vi "IRH1-2T_ConstructiveHeuristic.vi"(9 "Initial Construction Heursitic":T1, 10 "Scheduler":T2(ring)=enum."Non Delay Scheduler", 11 "Proocessing Times MxJ":u16[][](array[numeric])=[[1, 69, 192, 47, 292, 28, 166, 205], [146, 96, 177, 62, 37, 145, 3, 334], [99, 182, 133, 113, 9, 239, 27, 198], [159, 182, 132, 158, 183, 38, 142, 6], [92, 63, 114, 144, 180, 199, 136, 72], [119, 31, 9, 163, 139, 158, 350, 31], [46, 30, 59, 290, 156, 90, 175, 154], [338, 347, 184, 23, 4, 103, 1, 0]]) -> (1 "Due Dates":u16[](array[numeric]), 2 "Total Tardiness":i32, 3 "IRH2T Schedule Out":u16[](array[numeric]))   [LabVIEW 2013]
uses:
  Initial Construction Heuristic.ctl
  Classes/GanntChart.lvclass
panel:
  in  "Proocessing Times (8x8)":u16[][](array[numeric])=[[1, 69, 192, 47, 292, 28, 166, 205], [146, 96, 177, 62, 37, 145, 3, 334], [99, 182, 133, 113, 9, 239, 27, 198], [159, 182, 132, 158, 183, 38, 142, 6], [92, 63, 114, 144, 180, 199, 136, 72], [119, 31, 9, 163, 139, 158, 350, 31], [46, 30, 59, 290, 156, 90, 175, 154], [338, 347, 184, 23, 4, 103, 1, 0]]
  out "Machine Completion Times":u16[](array[numeric])
  out "Completion Times":u16[][](array[numeric])
  out "Job Completion Times":i32[](array[numeric])
  out "String":string
  out "LPT Array":i32[](array[numeric])
  # "1, 69, 192, 47, 292, 28, 166, 205], \n[146, 96, 177, 62, 37, 145, 3, 334], \n[99, 182, 133, 113, 9, 239, 27, 198], \n[159, 182, 132, 158, 183, 38, 142, 6], \n[92, 63, 114, 144, 180, 199, 136, 72], \n[119, 31, 9, 163, 139, 158, 350, 31], \n[46, 30, 59, 290, 156, 90, 175, 154], \n[338, 347, 184, 23, 4, 103, 1, 0]]"
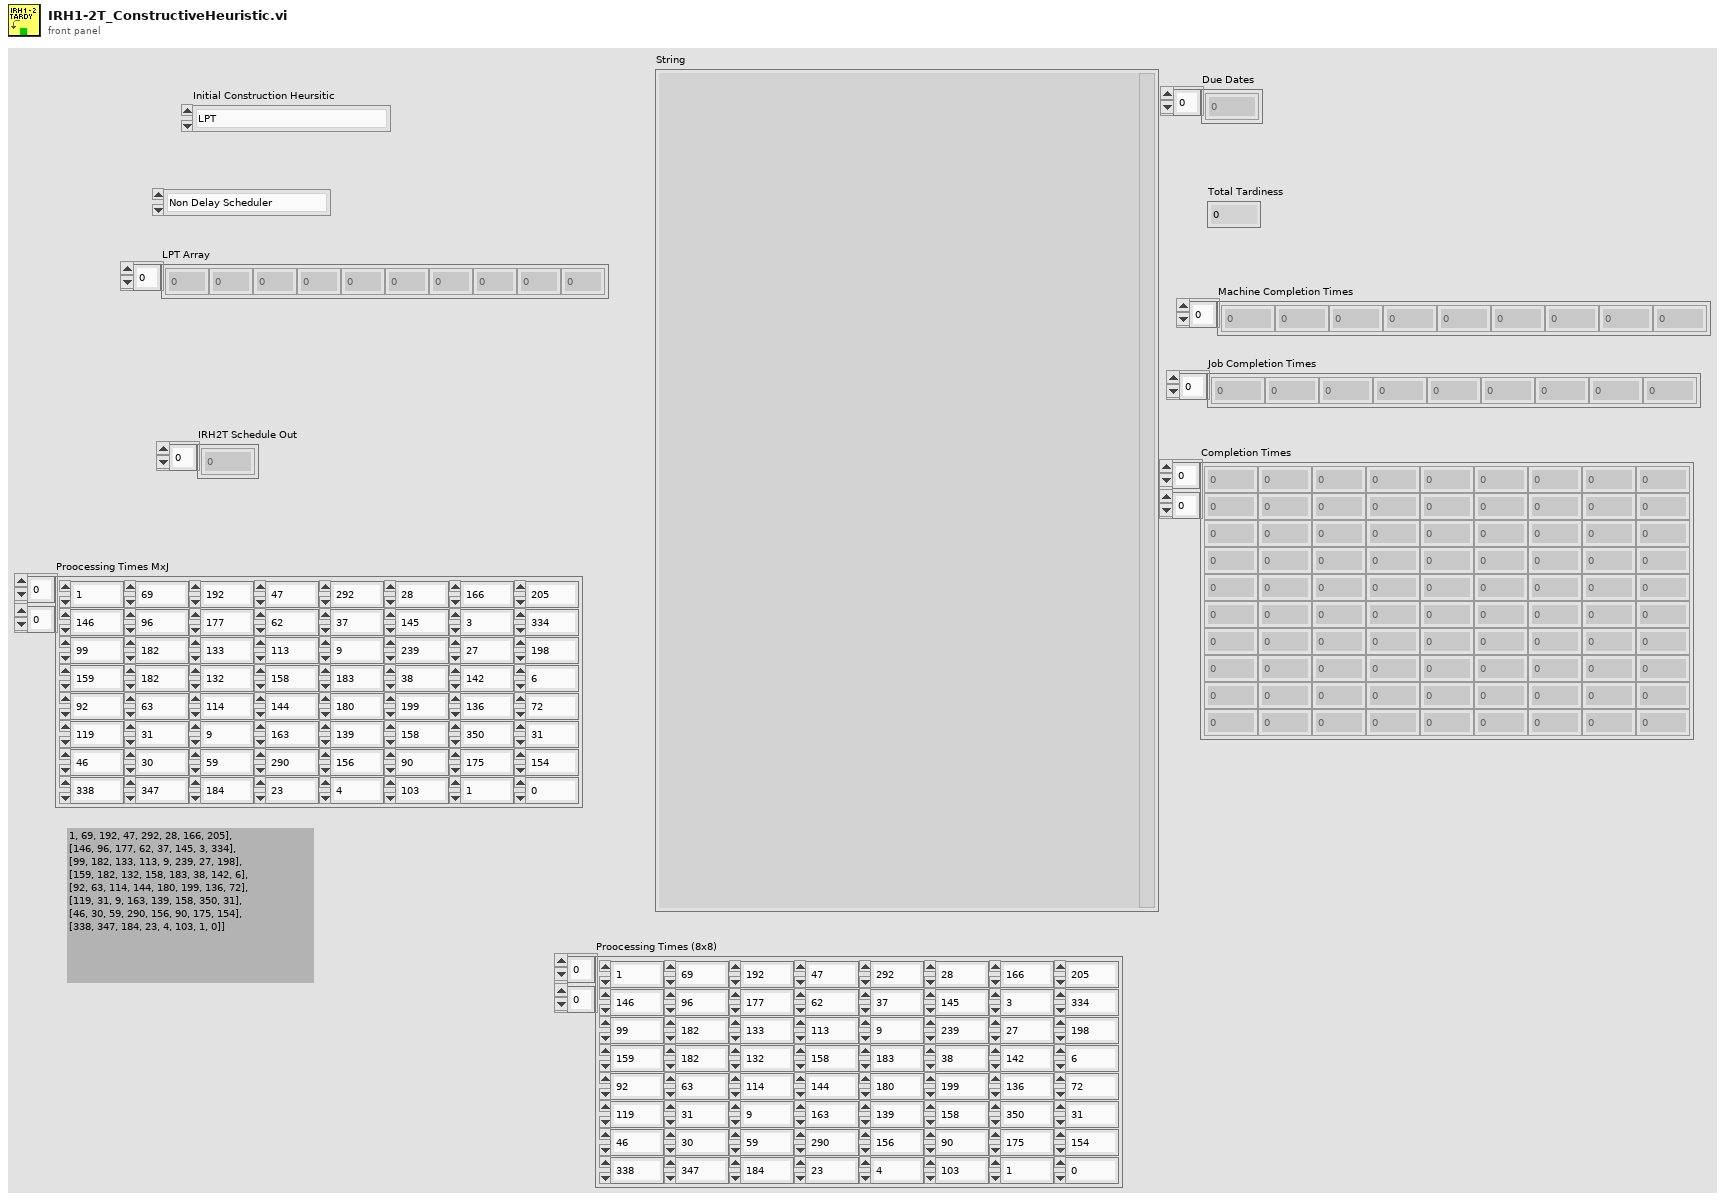
[diagram p1: front panel]
types:
  T1 = typedef "Initial Construction Heuristic.ctl" = enum16{"LPT", "SPT", "EDD"}
  T2 = enum16{"Semi Active Scheduler", "Non Delay Scheduler"}
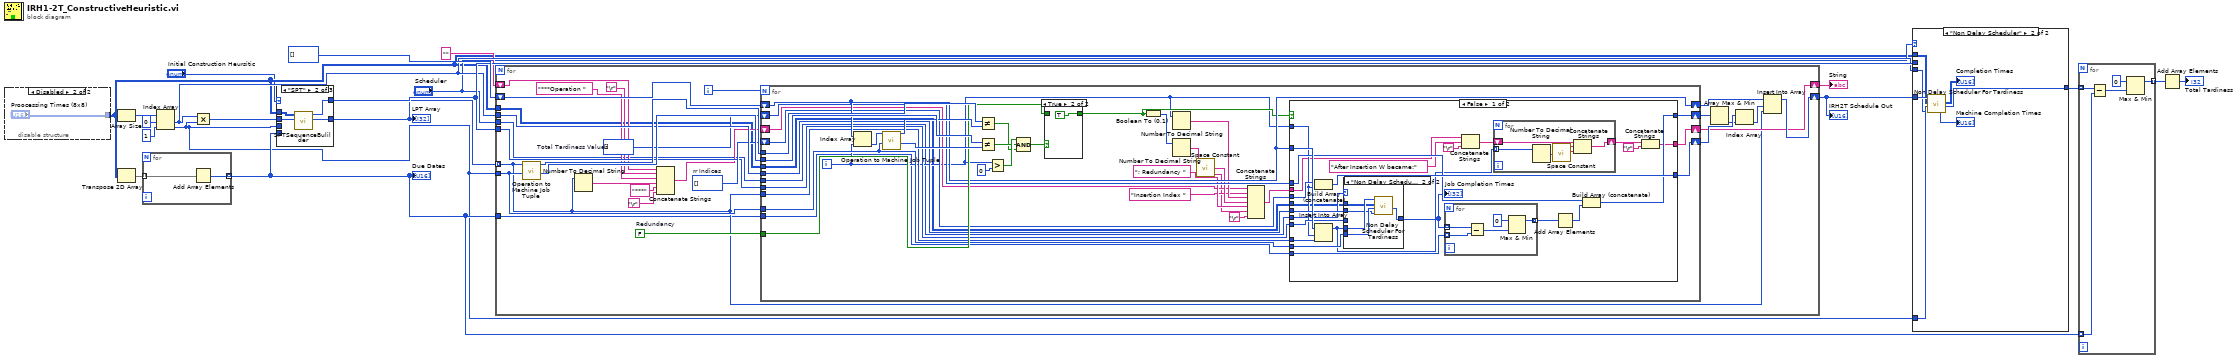
[diagram p0: block diagram]
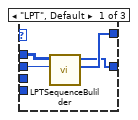
[diagram p2: hidden frame]
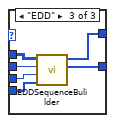
[diagram p3: hidden frame]
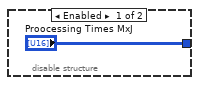
[diagram p4: hidden frame]
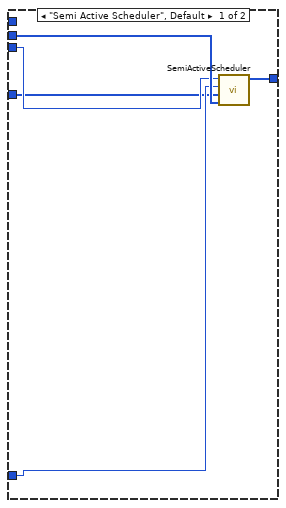
[diagram p5: hidden frame]
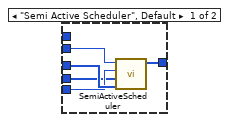
[diagram p6: hidden frame]
diagram:
  n1 = disable-structure shown="Disabled" {
    disable-tunnel: ["Proocessing Times MxJ" "Proocessing Times (8x8)"] -> w4
    frame Enabled {
    }
    frame Disabled {
    }
  }
  n2 = Array Size(array=w4) -> (size(s)=w20:i32[])
  n3 = Transpose 2D Array(2D array=w4) -> (transposed array=w10:u16[][])
  n4 = for {
    tunnel: w10 -> [w24] mode=indexing
    tunnel: [w23] -> w2 mode=indexing
    n5 = Add Array Elements(numeric array=w24) -> (sum=w23:u16)
  }
  "Due Dates" <- w2
  n6 = Index Array(array=w20, index #1=0 ("index"), index #2=1 ("index")) -> (element #1=w15:i32, element #2=w1:i32)
  n7 = Multiply(x=w15, y=w1) -> (x*y=w5:i32)
  n8 = case shown="\"SPT\"" "Initial Construction Heursitic" {
    tunnel: [w28 w30 w36] -> w16
    tunnel: [w27 w29 w35] -> w11
    tunnel: w5 -> [w26 w31 w37]
    tunnel: w4 -> [w25 w32 w38]
    tunnel: w2 -> [_ _ w33]
    tunnel: w1 -> [_ _ w34]
    frame "LPT", Default {
      n9 = call "LPTSequenceBulilder.vi"("Number Of Operations"=w26, "Proocessing Times MxJ"=w25) -> ("Falttened Processing Times"=w28:u16[], "LPT Sequence"=w27:i32[])  [unwired: 8 in]
    }
    frame "SPT" {
      n10 = call "SPTSequenceBulilder.vi"("Number Of Operations"=w31, "Proocessing Times MxJ"=w32) -> ("SPT Sequence"=w29:i32[], "Flattened Processing Times"=w30:u16[])  [unwired: 8 in]
    }
    frame "EDD" {
      n11 = call "EDDSequenceBulilder.vi"("Due Dates"=w33, "Number Of Machines"=w34, "Number Of Operations"=w37, "Proocessing Times MxJ"=w38) -> ("EDD Squence"=w35:i32[], "Flattened Processing Times"=w36:u16[])  [unwired: 6 in]
    }
  }
  "LPT Array" <- w11
  n12 = for {
    tunnel: w11 -> [w48] mode=indexing
    tunnel: w1 -> [w60]
    shift-right: [w52] -> w6
    shift-left: u16[] [] -> [w64]
    tunnel: w16 -> [w53]
    tunnel: w15 -> [w59]
    shift-right: [w50] -> w13
    shift-left: "" -> [w49]
    tunnel: w4 -> [w41]
    tunnel: "Scheduler" -> [w40]
    tunnel: w2 -> [w39]
    i -> [w66]
    w57 = i32[] []  # Total Tardiness Values
    w58 = i32[] []  # rr Indices
    w65 = FALSE  # Redundancy
    n13 = call "Operation to Machine Job Tuple.vi"("Number of Machines"=w60, "Operation Number"=w48) -> ("Job No"=w61:i32, "Machine No"=w62:i32)  [unwired: 8 in]
    n14 = Number To Decimal String(number=w48) -> (decimal integer string=w46:string)  [unwired: 1 in]
    n15 = Concatenate Strings(w49, "\r", "***Operation " ("string"), w46, "***" ("string"), "\r") -> (w45:string)
    n16 = for {
      N: w66 -> [_]
      shift-right: [w92] -> w63
      shift-left: w64 -> [w92]
      tunnel: w62 -> [w96]
      tunnel: w61 -> [w99]
      tunnel: w60 -> [w89]
      tunnel: w65 -> [w93]
      tunnel: w48 -> [w91]
      tunnel: w53 -> [w90]
      tunnel: w59 -> [w88]
      shift-right: [w86] -> w56
      shift-left: w58 -> [w87]
      shift-right: [w84] -> w51
      shift-left: w57 -> [w85]
      shift-right: [w82] -> w50
      shift-left: w45 -> [w76]
      tunnel: w41 -> [w69]
      tunnel: w40 -> [w68]
      tunnel: w39 -> [w67]
      i -> [w73]
      n17 = Index Array(array=w92, index=w73) -> (element=w81:u16)
      n18 = call "Operation to Machine Job Tuple.vi"("Number of Machines"=w89, "Operation Number"=w81) -> ("Job No"=w98:i32, "Machine No"=w95:i32)  [unwired: 8 in]
      n19 = Not Equal?(x=w96, y=w95) -> (x != y?=w83:bool)
      n20 = Not Equal?(x=w99, y=w98) -> (x != y?=w97:bool)
      n21 = Greater?(x=w73, y=0) -> (0:w100:bool)
      n22 = Compound Arithmetic op=AND(w100, w97, w83) -> (w94:bool)
      n23 = case shown="True" w94 {
        tunnel: w93 -> [w149 _]
        tunnel: [w149 TRUE ("Redundancy")] -> w74
        frame False {
        }
        frame True {
        }
      }
      n24 = Boolean To (0,1)(Boolean=w74) -> (0, 1=w72:i16)
      n25 = Number To Decimal String(number=w73) -> (decimal integer string=w78:string)  [unwired: 1 in]
      n26 = Number To Decimal String(number=w72) -> (decimal integer string=w71:string)  [unwired: 1 in]
      n27 = call <vilib>:"Space Constant.vi"() -> ("String"=w79:string)
      n28 = Concatenate Strings(w76, "Insertion Index " ("string"), w78, w79, "; Redundancy " ("string"), w71, "\r") -> (w75:string)
      n29 = case shown="False" w74 {
        tunnel: w92 -> [w125 _]
        tunnel: w91 -> [w124 _]
        tunnel: w90 -> [w123 _]
        tunnel: w89 -> [w122 _]
        tunnel: w88 -> [w121 _]
        tunnel: w87 -> [w120 w148]
        tunnel: w73 -> [w114 _]
        tunnel: [w119 w148] -> w86
        tunnel: w85 -> [w118 w147]
        tunnel: [w117 w147] -> w84
        tunnel: [w115 w146] -> w82
        tunnel: w75 -> [w113 w146]
        tunnel: w69 -> [w106 _]
        tunnel: w68 -> [w107 _]
        tunnel: w67 -> [w104 _]
        frame False {
          n30 = Build Array (concatenate)(w120, w114) -> (w119:i32[])
          n31 = Insert Into Array(array=w125, index=w114, new element=w124) -> (w116:u16[])
          n32 = case shown="\"Non Delay Scheduler\"" w107 {
            tunnel: w123 -> [w135 _]
            tunnel: w122 -> [w134 w139]
            tunnel: w121 -> [w133 w138]
            tunnel: [w132 w137] -> w105
            tunnel: w116 -> [w131 w140]
            tunnel: w106 -> [_ w136]
            frame "Semi Active Scheduler", Default {
              n33 = call "SemiActiveScheduler.vi"("Proocessing Times"=w135, "Schedule"=w131, "Number Of Machines"=w134, "Number Of Jobs"=w133) -> ("Job Completion Times"=w132:i32[])  [unwired: 5 in, 2 out]
            }
            frame "Non Delay Scheduler" {
              n34 = call "Non Delay Scheduler For Tardiness.vi"("Number of  Jobs"=w138, "Number of Machines"=w139, "Processing Times"=w136, "Schedule"=w140) -> ("Job Completion Times"=w137:u16[])  [unwired: 3 in, 4 out]
            }
          }
          "Job Completion Times" <- w105
          n35 = for {
            tunnel: w105 -> [w130] mode=indexing
            tunnel: w104 -> [w129] mode=indexing
            tunnel: [w126] -> w103 mode=indexing
            n36 = Subtract(x=w130, y=w129) -> (x-y=w128:i32)
            n37 = Max & Min(x=0, y=w128) -> (max(x,y)=w126:i32)  [unwired: 1 out]
          }
          n38 = Concatenate Strings(w113, "After Insertion W became:" ("string"), "\r") -> (w110:string)
          n39 = for {
            tunnel: w116 -> [w145] mode=indexing
            shift-right: [w142] -> w109
            shift-left: w110 -> [w144]
            n40 = Number To Decimal String(number=w145) -> (decimal integer string=w143:string)  [unwired: 1 in]
            n41 = call <vilib>:"Space Constant.vi"() -> ("String"=w141:string)
            n42 = Concatenate Strings(w144, w143, w141) -> (w142:string)
          }
          n43 = Add Array Elements(numeric array=w103) -> (sum=w102:i32)
          n44 = Build Array (concatenate)(w118, w102) -> (w117:i32[])
          n45 = Concatenate Strings(w109, "\r") -> (w115:string)
        }
        frame True {
        }
      }
    }
    n46 = Array Max & Min(array=w51) -> (min index (indices)=w55:i32)  [unwired: 3 out]
    n47 = Index Array(array=w56, index=w55) -> (element=w54:i32)
    n48 = Insert Into Array(array=w63, index=w54, new element=w48) -> (w52:u16[])
  }
  "String" <- w13
  "IRH2T Schedule Out" <- w6
  n49 = case shown="\"Non Delay Scheduler\"" "Scheduler" {
    tunnel: w6 -> [w151 w162]
    tunnel: w16 -> [w155 _]
    tunnel: w1 -> [w154 w161]
    tunnel: w15 -> [w153 w160]
    tunnel: [w152 w159] -> w9
    tunnel: w4 -> [_ w156]
    frame "Semi Active Scheduler", Default {
      n50 = call "SemiActiveScheduler.vi"("Proocessing Times"=w155, "Schedule"=w151, "Number Of Machines"=w154, "Number Of Jobs"=w153) -> ("Job Completion Times"=w152:i32[])  [unwired: 5 in, 2 out]
    }
    frame "Non Delay Scheduler" {
      n51 = call "Non Delay Scheduler For Tardiness.vi"("Number of  Jobs"=w160, "Number of Machines"=w161, "Processing Times"=w156, "Schedule"=w162) -> ("Job Completion Times"=w159:u16[], "Completion Times"=→"Completion Times":u16[][], "Machine Completion Times"=→"Machine Completion Times":u16[])  [unwired: 3 in, 2 out]
    }
  }
  n52 = for {
    tunnel: w9 -> [w167] mode=indexing
    tunnel: w2 -> [w166] mode=indexing
    tunnel: [w163] -> w8 mode=indexing
    n53 = Subtract(x=w167, y=w166) -> (x-y=w165:i32)
    n54 = Max & Min(x=0, y=w165) -> (max(x,y)=w163:i32)  [unwired: 1 out]
  }
  n55 = Add Array Elements(numeric array=w8) -> (sum=→"Total Tardiness":i32)
